vi "SendOutput.vi"(8 "error in (no error)":errorcluster, 11 "Subsystem in":refnum<class "Subsystem.lvclass">) -> (0 "error out":errorcluster, 3 "Subsystem out":refnum<class "Subsystem.lvclass">)   [LabVIEW 2017, in "Subsystem.lvclass"]
uses:
  Subsystem.lvclass
  Subsystem.lvclass/Subsystem.ctl
  SubsystemData/SubsystemData.lvclass
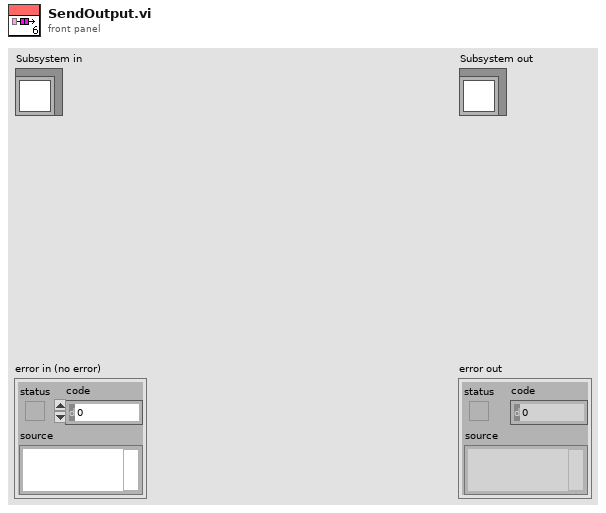
[diagram p1: front panel]
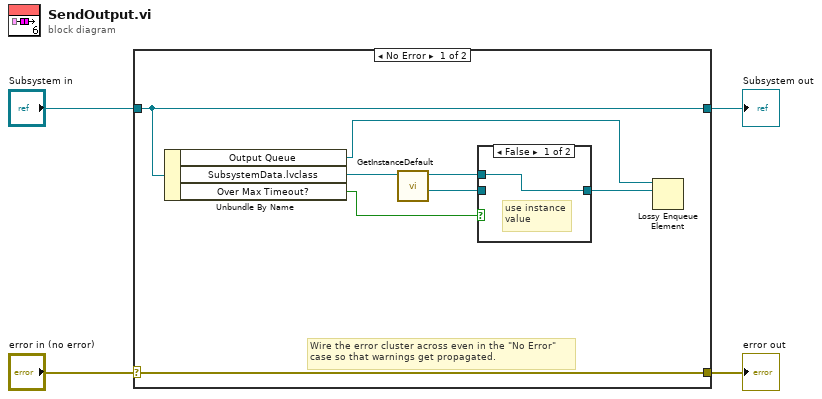
[diagram p0: block diagram]
diagram:
  n1 = case shown="No Error" "error in (no error)" {
    selector: "error in (no error)" -> [w12 w16]
    tunnel: [w12 w16] -> w3
    tunnel: [w11 w15] -> w1
    tunnel: "Subsystem in" -> [w11 w15]
    frame No Error {
      # "Wire the error cluster across even in the \"No Error\"\ncase so that warnings get propagated."
      n2 = Unbundle By Name(w11) -> ("Output Queue"=w5:refnum<queue>, "SubsystemData.lvclass"=w7:refnum<class "SubsystemData.lvclass">, "Over Max Timeout?"=w8:bool)
      n3 = call-dynamic "GetInstanceDefault.vi"("Subsystem in"=w7) -> ("Instance Default"=w9:refnum<class "SubsystemData.lvclass">, "Subsystem out"=w10:refnum<class "SubsystemData.lvclass">)  [unwired: 8 in, 1 out]
      n4 = case shown="False" w8 {
        tunnel: w10 -> [w13 _]
        tunnel: w9 -> [_ w14]
        tunnel: [w13 w14] -> w6
        frame False {
          # "use instance\nvalue"
        }
        frame True {
          # "use instance\nclass default"
        }
      }
      n5 = Lossy Enqueue Element(queue=w5, element=w6) -> ()  [unwired: 1 in, 4 out]
    }
    frame Error {
    }
  }
  "error out" <- w3
  "Subsystem out" <- w1
